vi "Update UI.vi"(8 "error in (no error)":errorcluster, 10 "Image In":T1, 11 "Camera Prime95B Controller in":refnum<class "Camera Prime95B Controller.lvclass">) -> (0 "error out":errorcluster, 3 "Camera Prime95B Controller out":refnum<class "Camera Prime95B Controller.lvclass">)   [LabVIEW 2020, in "Camera_Prime95B.lvlib" / "Camera Prime95B Controller.lvlib" / "Camera Prime95B Controller.lvclass"]
uses:
  Camera Prime95B Controller.lvclass
  <vilib>/vision/Image Controls.llb/IMAQ Image.ctl
  Camera Prime95B Controller.lvclass/Camera Prime95B Controller.ctl
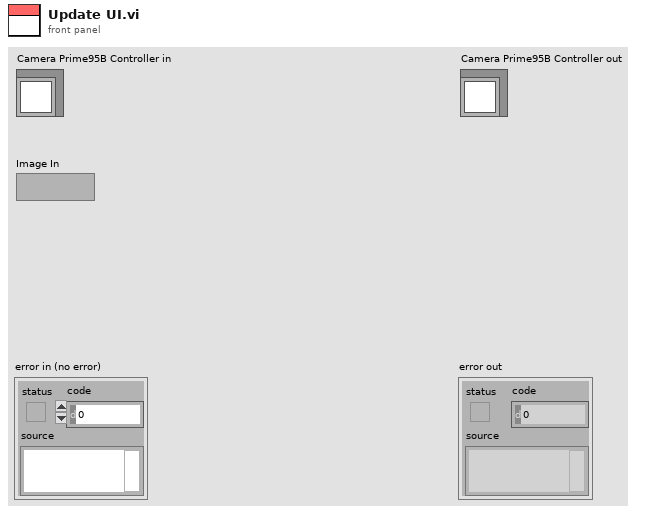
[diagram p1: front panel]
types:
  T1 = typedef "IMAQ Image.ctl" = refnum<image>
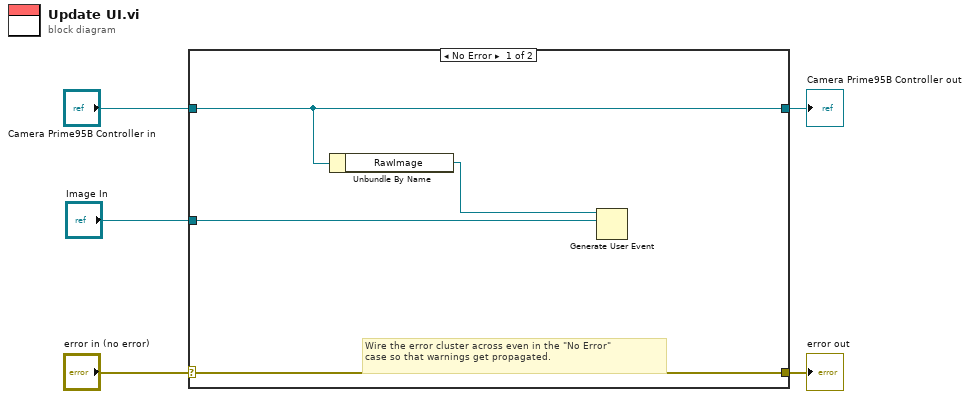
[diagram p0: block diagram]
diagram:
  n1 = case shown="No Error" "error in (no error)" {
    selector: "error in (no error)" -> [w9 w11]
    tunnel: [w9 w11] -> w4
    tunnel: [w8 w10] -> w2
    tunnel: "Camera Prime95B Controller in" -> [w8 w10]
    tunnel: "Image In" -> [w6 _]
    frame No Error {
      # "Wire the error cluster across even in the \"No Error\"\ncase so that warnings get propagated."
      n2 = Unbundle By Name(w8) -> ("RawImage"=w7:refnum<user-event>)
      n3 = Generate User Event(user event=w7, event data cluster=w6) -> ()  [unwired: 2 in, 2 out]
    }
    frame Error {
    }
  }
  "error out" <- w4
  "Camera Prime95B Controller out" <- w2
